vi "BINARIOS.vi"() -> ()   [LabVIEW 2013]
panel:
  out "Cantidad Disminuye":dbl
  out "BINARIO":bool[](array[boolean])
  out "Cantidad Aumenta":dbl
  # "UNIVERSIDAD DE CUNDIMARCA\nINGENIERIA DE SISTEMAS\nANDY CAMARGO\nRAFAEL REYES \nELECTIVA PROFESIONAL IV"
  # "1"
  # "2"
  # "4"
  # "8"
  # "16"
  # "32"
  # "64"
  # "128"
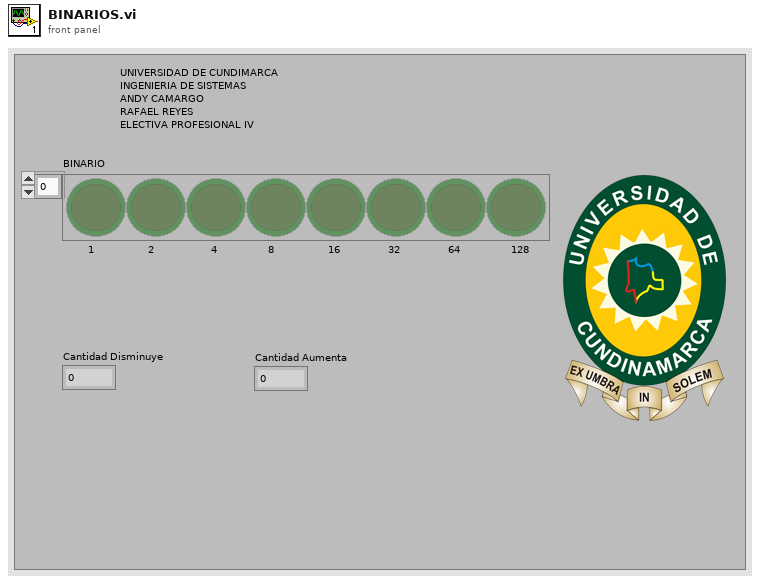
[diagram p1: front panel]
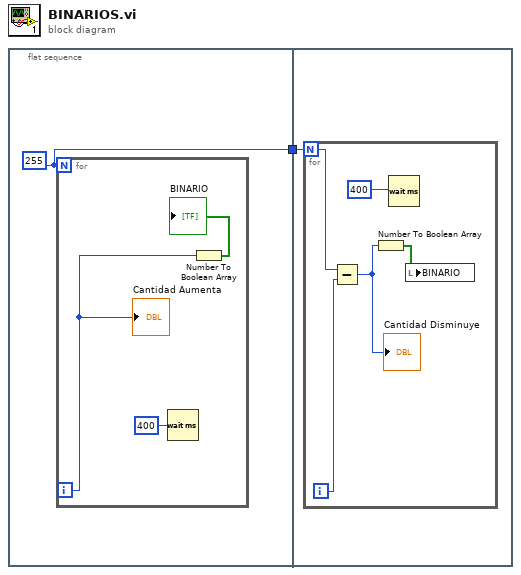
[diagram p0: block diagram]
diagram:
  n1 = flat-sequence {
    tunnel: [w2] -> w1
    tunnel: w1 -> [w6]
    frame #0 {
      w2 = 255
      n2 = for {
        N: w2 -> [_]
        i -> [w3]
        n3 = Wait (ms)(milliseconds to wait=u32 400) -> ()  [unwired: 1 out]
        n4 = Number To Boolean Array(number=w3) -> (Boolean array=→"BINARIO":bool[])
        "Cantidad Aumenta" <- w3
      }
    }
    frame #1 {
      n5 = for {
        N: w6 -> [w10]
        i -> [w11]
        n6 = Subtract(x=w10, y=w11) -> (x-y=w8:i32)
        "Cantidad Disminuye" <- w8
        n7 = Number To Boolean Array(number=w8) -> (Boolean array=w9:bool[])
        n8 = Wait (ms)(milliseconds to wait=u32 400 ("millisecond timer value")) -> ()  [unwired: 1 out]
        n9 = local write "BINARIO"(w9) -> ()
      }
    }
  }
